vi "Handle Unit.vi"(5 "BTeam in":refnum<class "BTeam.lvclass">, 7 "p[x][y]":i32[][](array[numeric]), 9 "Player[p] in":T1[](array[typedef]), 11 "Unit in":T6) -> (1 "Player[p] out":T1[](array[typedef]), 3 "Unit out":T6)   [LabVIEW 2015, in "BTeam.lvclass"]
uses:
  BTeam.lvclass
  Team Cluster.ctl
  Mode Enum.ctl
  TeamEffort/private/Player Cluster.ctl
  Square/Square.lvclass
  TeamEffort/Team Move Input.ctl
  Type Defs/Action Enum.ctl
  TeamEffort/Team Move Output.ctl
  Type Defs/Direction Enum.ctl
  Type Defs/SB Type Defs.lvlib
  TeamEffort/TeamEffort.lvclass
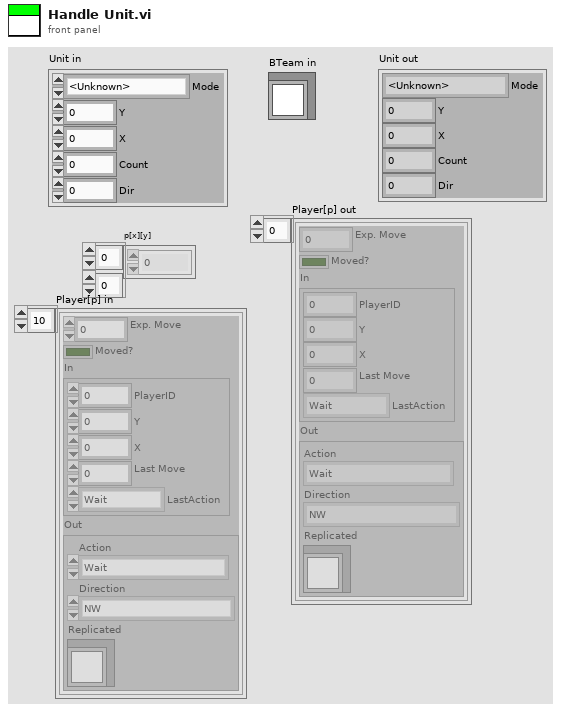
[diagram p1: front panel]
types:
  T1 = typedef "TeamEffort.lvclass/Player Cluster.ctl" = cluster{"Exp. Move":i32, "Moved?":bool, "In":T2, "Out":T4}
  T2 = typedef "TeamEffort.lvclass/Team Move Input.ctl" = cluster{"PlayerID":i32, "Y":i32, "X":i32, "Last Move":i32, "LastAction":T3}
  T3 = typedef "SB Type Defs.lvlib/Action Enum.ctl" = enum16{"Wait", "Move", "Attack", "Replicate"}
  T4 = typedef "TeamEffort.lvclass/Team Move Output.ctl" = cluster{"Action":T3, "Direction":T5, "Replicated":refnum<class "Square.lvclass">}
  T5 = typedef "SB Type Defs.lvlib/Direction Enum.ctl" = enum16{"NW", "N", "NE", "E", "SE", "S", "SW", "W"}
  T6 = typedef "BTeam.lvclass/Team Cluster.ctl" = cluster{"Mode":T7, "Y":i32, "X":i32, "Count":i32, "Dir":i32}
  T7 = typedef "BTeam.lvclass/Mode Enum.ctl" = enum16{"<Unknown>", "1", "2", "4", "8", "16", "Check", "Spawn"}
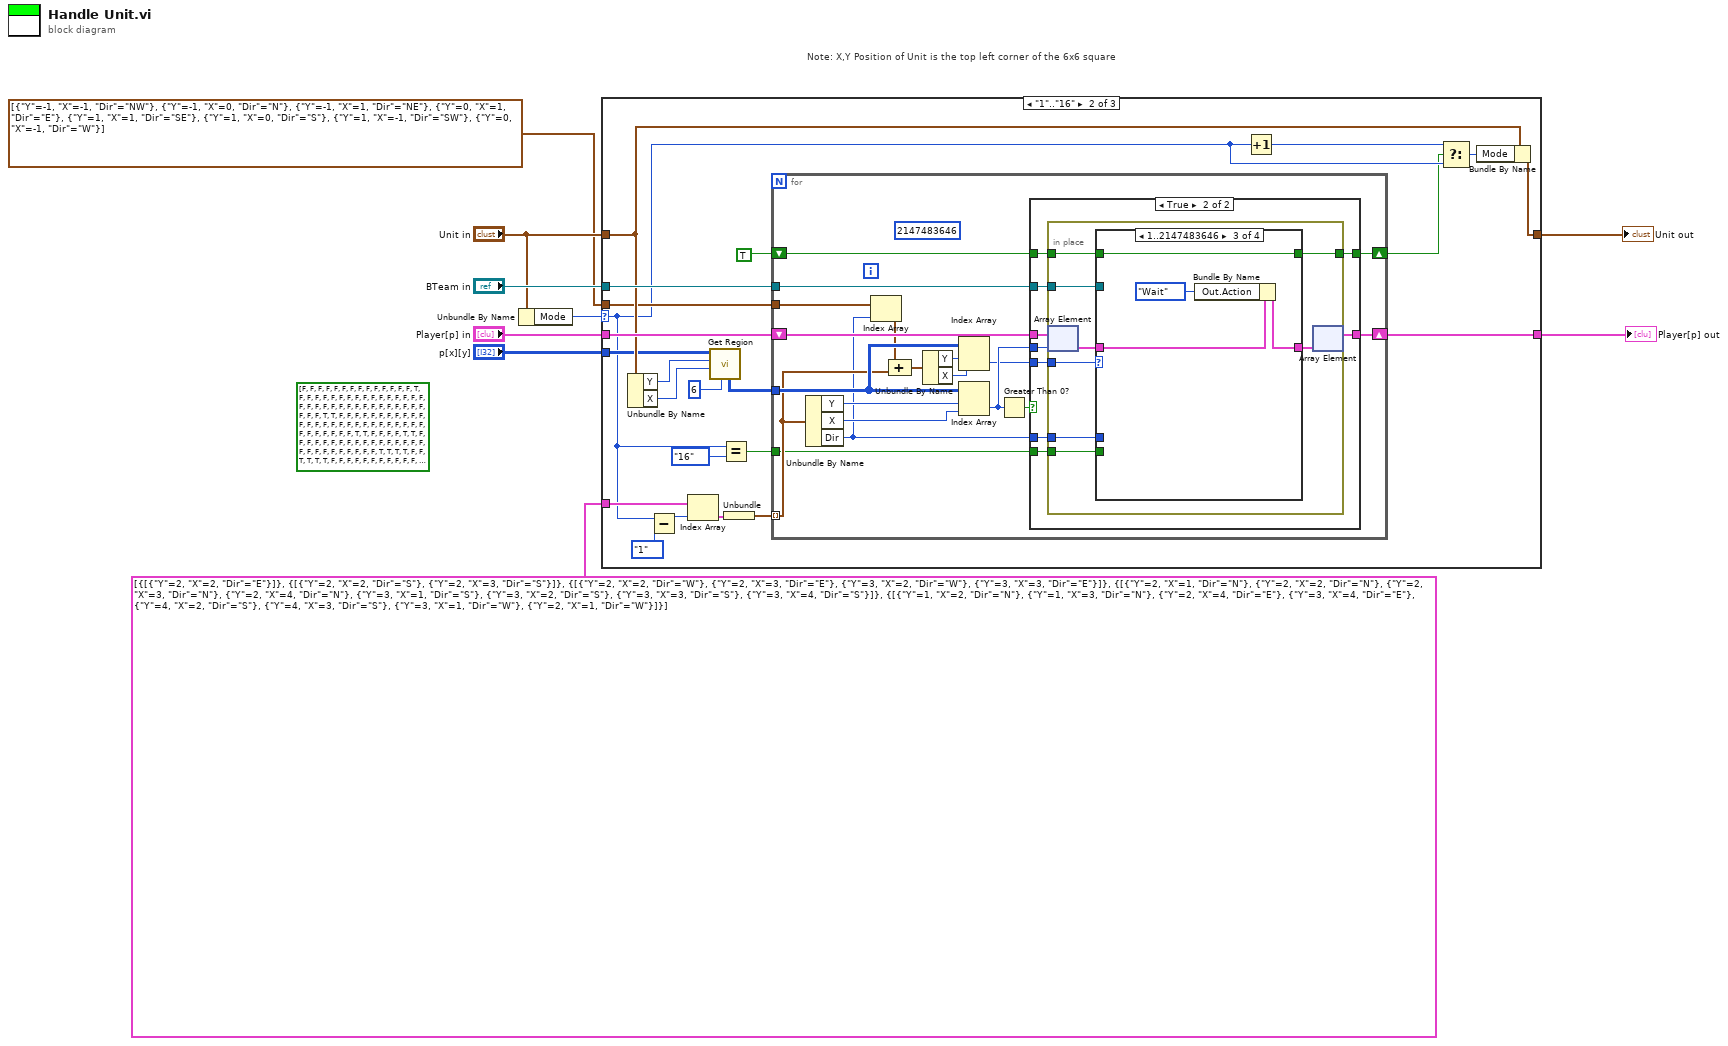
[diagram p0: block diagram]
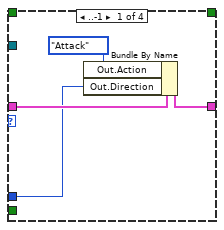
[diagram p4: hidden frame]
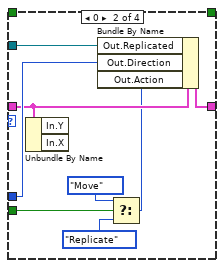
[diagram p5: hidden frame]
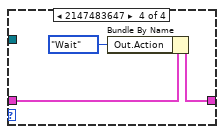
[diagram p6: hidden frame]
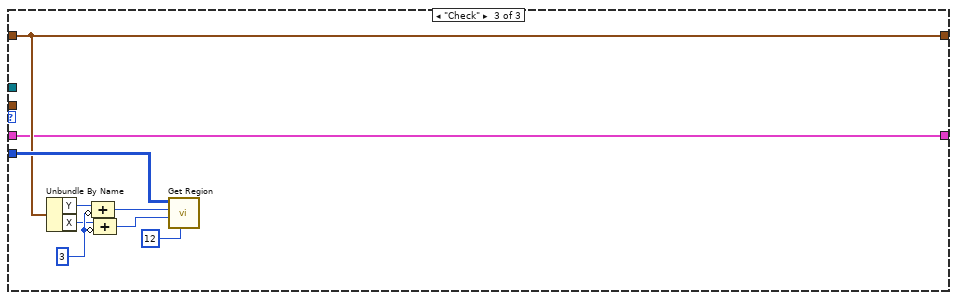
[diagram p7: hidden frame]
diagram:
  (unwired) bool[][][] [[[FALSE, FALSE, FALSE, FALSE, FALSE, FALSE], [FALSE, FALSE, FALSE, FALSE, FALSE, FALSE], [FALSE, FALSE, TRUE, FALSE, FALSE, FALSE], [FALSE, FALSE, FALSE, FALSE, FALSE, FALSE], [FALSE, FALSE, FALSE, FALSE, FALSE, FALSE], [FALSE, FALSE, FALSE, FALSE, FALSE, FALSE]], [[FALSE, FALSE, FALSE, FALSE, FALSE, FALSE], [FALSE, FALSE, FALSE, FALSE, FALSE, FALSE], [FALSE, FALSE, TRUE, TRUE, FALSE, FALSE], [FALSE, FALSE, FALSE, FALSE, FALSE, FALSE], [FALSE, FALSE, FALSE, FALSE, FALSE, FALSE], [FALSE, FALSE, FALSE, FALSE, FALSE, FALSE]], [[FALSE, FALSE, FALSE, FALSE, FALSE, FALSE], [FALSE, FALSE, FALSE, FALSE, FALSE, FALSE], [FALSE, FALSE, TRUE, TRUE, FALSE, FALSE], [FALSE, FALSE, TRUE, TRUE, FALSE, FALSE], [FALSE, FALSE, FALSE, FALSE, FALSE, FALSE], [FALSE, FALSE, FALSE, FALSE, FALSE, FALSE]], [[FALSE, FALSE, FALSE, FALSE, FALSE, FALSE], [FALSE, FALSE, FALSE, FALSE, FALSE, FALSE], [FALSE, TRUE, TRUE, TRUE, TRUE, FALSE], [FALSE, TRUE, TRUE, TRUE, TRUE, FALSE], [FALSE, FALSE, FALSE, FALSE, FALSE, FALSE], [FALSE, FALSE, FALSE, FALSE, FALSE, FALSE]], [[FALSE, FALSE, FALSE, FALSE, FALSE, FALSE], [FALSE, TRUE, TRUE, TRUE, TRUE, FALSE], [FALSE, TRUE, TRUE, TRUE, TRUE, FALSE], [FALSE, TRUE, TRUE, TRUE, TRUE, FALSE], [FALSE, TRUE, TRUE, TRUE, TRUE, FALSE], [FALSE, FALSE, FALSE, FALSE, FALSE, FALSE]], [[FALSE, FALSE, TRUE, TRUE, FALSE, FALSE], [FALSE, TRUE, FALSE, FALSE, TRUE, FALSE], [TRUE, FALSE, TRUE, TRUE, FALSE, TRUE], [TRUE, FALSE, TRUE, TRUE, FALSE, TRUE], [FALSE, TRUE, FALSE, FALSE, TRUE, FALSE], [FALSE, FALSE, TRUE, TRUE, FALSE, FALSE]]]
  # "Note: X,Y Position of Unit is the top left corner of the 6x6 square"
  n1 = Unbundle By Name("Unit in") -> ("Mode"=w5:T7)
  n2 = case shown="\"1\"..\"16\"" w5 {
    selector: w5 -> [_ w14 _]
    tunnel: "Player[p] in" -> [w11 w34 w92]
    tunnel: [w11 w33 w92] -> w7
    tunnel: "p[x][y]" -> [_ w29 w99]
    tunnel: "BTeam in" -> [_ w32 _]
    tunnel: "Unit in" -> [w10 w30 w93]
    tunnel: [w10 w31 w93] -> w3
    tunnel: cluster{cluster{"Y":i32, "X":i32, "Dir":T5}[]}[] [{[{"Y"=2, "X"=2, "Dir"=enum."E"}]}, {[{"Y"=2, "X"=2, "Dir"=enum."S"}, {"Y"=2, "X"=3, "Dir"=enum."S"}]}, {[{"Y"=2, "X"=2, "Dir"=enum."W"}, {"Y"=2, "X"=3, "Dir"=enum."E"}, {"Y"=3, "X"=2, "Dir"=enum."W"}, {"Y"=3, "X"=3, "Dir"=enum."E"}]}, {[{"Y"=2, "X"=1, "Dir"=enum."N"}, {"Y"=2, "X"=2, "Dir"=enum."N"}, {"Y"=2, "X"=3, "Dir"=enum."N"}, {"Y"=2, "X"=4, "Dir"=enum."N"}, {"Y"=3, "X"=1, "Dir"=enum."S"}, {"Y"=3, "X"=2, "Dir"=enum."S"}, {"Y"=3, "X"=3, "Dir"=enum."S"}, {"Y"=3, "X"=4, "Dir"=enum."S"}]}, {[{"Y"=1, "X"=2, "Dir"=enum."N"}, {"Y"=1, "X"=3, "Dir"=enum."N"}, {"Y"=2, "X"=4, "Dir"=enum."E"}, {"Y"=3, "X"=4, "Dir"=enum."E"}, {"Y"=4, "X"=2, "Dir"=enum."S"}, {"Y"=4, "X"=3, "Dir"=enum."S"}, {"Y"=3, "X"=1, "Dir"=enum."W"}, {"Y"=2, "X"=1, "Dir"=enum."W"}]}] -> [_ w19 _]
    tunnel: cluster{"Y":i32, "X":i32, "Dir":T5}[] [{"Y"=-1, "X"=-1, "Dir"=enum."NW"}, {"Y"=-1, "X"=0, "Dir"=enum."N"}, {"Y"=-1, "X"=1, "Dir"=enum."NE"}, {"Y"=0, "X"=1, "Dir"=enum."E"}, {"Y"=1, "X"=1, "Dir"=enum."SE"}, {"Y"=1, "X"=0, "Dir"=enum."S"}, {"Y"=1, "X"=-1, "Dir"=enum."SW"}, {"Y"=0, "X"=-1, "Dir"=enum."W"}] -> [_ w16 _]
    frame "<Unknown>", Default {
    }
    frame "1".."16" {
      n3 = Unbundle By Name(w30) -> ("Y"=w28:i32, "X"=w27:i32)
      n4 = Subtract(x=w14, y=Mode_Enum."1") -> (x-y=w21:u16)
      n5 = Index Array(array=w19, index=w21) -> (element=w18:cluster{cluster{"Y":i32, "X":i32, "Dir":T5}[]})
      n6 = call "Get Region.vi"("size"=6, "X"=w27, "Y"=w28, "p[x][y]"=w29) -> ("Region out[12][12]"=w20:i32[][])  [unwired: 7 in]
      n7 = Equal?(x=w14, y=Mode_Enum."16") -> (x = y?=w13:bool)
      n8 = Unbundle(w18) -> (w17:cluster{"Y":i32, "X":i32, "Dir":T5}[])
      n9 = for {
        tunnel: w32 -> [w49]
        shift-right: [w52] -> w33
        shift-left: w34 -> [w53]
        tunnel: w20 -> [w44]
        shift-right: [w50] -> w12
        shift-left: TRUE -> [w51]
        tunnel: w17 -> [w42] mode=indexing
        tunnel: w16 -> [w41]
        tunnel: w13 -> [w35]
        (unwired) 2147483646 ("size")
        n10 = Unbundle By Name(w42) -> ("Y"=w46:i32, "X"=w45:i32, "Dir"=w36:T5)
        n11 = Index Array(array=w41, index=w36) -> (element=w40:cluster{"Y":i32, "X":i32, "Dir":T5})
        n12 = Compound Arithmetic op=unknown(w40, w42) -> (w39:cluster{"Y":i32, "X":i32, "Dir":u16})
        n13 = Unbundle By Name(w39) -> ("Y"=w38:i32, "X"=w37:i32)
        n14 = Index Array(array=w44, index (row)=w38, index (col)=w37) -> (element=w43:i32)
        n15 = Index Array(array=w44, index (row)=w46, index (col)=w45) -> (element=w48:i32)
        n16 = Greater Than 0?(x=w48) -> (x > 0?=w47:bool)
        n17 = case shown="True" w47 {
          tunnel: w53 -> [w55 w64]
          tunnel: [w55 w63] -> w52
          tunnel: w51 -> [w54 w60]
          tunnel: w48 -> [_ w62]
          tunnel: [w54 w57] -> w50
          tunnel: w49 -> [_ w61]
          tunnel: w36 -> [_ w59]
          tunnel: w43 -> [_ w58]
          tunnel: w35 -> [_ w56]
          frame False {
          }
          frame True {
            n18 = in-place {
              in-place-border: w61 -> [w66]
              in-place-border: w60 -> [w69]
              in-place-border: w59 -> [w67]
              in-place-border: w58 -> [w70]
              in-place-border: [w68] -> w57
              in-place-border: w56 -> [w65]
              n19 = in-place-array #1(w64, w62) -> (w72:T1)
              n20 = case shown="1..2147483646" w70 {
                tunnel: w72 -> [w76 w78 w86 w91]
                tunnel: [w73 w84 w88 w90] -> w71
                tunnel: w69 -> [_ _ w85 _]
                tunnel: [_ _ w85 _] -> w68
                tunnel: w67 -> [w74 w82 _ _]
                tunnel: w66 -> [_ w83 _ _]
                tunnel: w65 -> [_ w81 _ _]
                frame ..-1 {
                  n21 = Bundle By Name(cluster=w76, "Out.Action"=Action_Enum."Attack", "Out.Direction"=w74) -> (w73:T1)
                }
                frame 0 {
                  n22 = Unbundle By Name(w78) -> ()  [unwired: 2 out]
                  n23 = Select(t=Action_Enum."Move" ("Out.Action"), s=w81, f=Action_Enum."Replicate" ("Out.Action")) -> (s? t:f=w77:T3)
                  n24 = Bundle By Name(cluster=w78, "Out.Replicated"=w83, "Out.Direction"=w82, "Out.Action"=w77) -> (w84:T1)
                }
                frame 1..2147483646 {
                  n25 = Bundle By Name(cluster=w86, "Out.Action"=Action_Enum."Wait") -> (w88:T1)
                }
                frame 2147483647 {
                  n26 = Bundle By Name(cluster=w91, "Out.Action"=Action_Enum."Wait") -> (w90:T1)
                }
              }
              n27 = in-place-array #1(w71) -> (w63:T1[])  [unwired: 1 out]
            }
          }
        }
      }
      n28 = Increment(x=w14) -> (x+1=w23:T7)
      n29 = Select(t=w23, s=w12, f=w14) -> (s? t:f=w22:T7)
      n30 = Bundle By Name(cluster=w30, "Mode"=w22) -> (w31:T6)
    }
    frame "Check" {
      w96 = 3 ("size")
      n31 = Unbundle By Name(w93) -> ("Y"=w98:i32, "X"=w95:i32)
      n32 = Compound Arithmetic op=ADD(w98, invert w96) -> (w97:i32)
      n33 = Compound Arithmetic op=ADD(w95, invert w96) -> (w94:i32)
      n34 = call "Get Region.vi"("size"=12, "X"=w94, "Y"=w97, "p[x][y]"=w99) -> ()  [unwired: 7 in, 1 out]
    }
  }
  "Unit out" <- w3
  "Player[p] out" <- w7
